vi "鼠标位置.vi"() -> ()   [LabVIEW 2015]
panel:
  out "索引":i32
  out "数组":dbl[][](array[numeric])
  in  "停止":bool
  out "垂直":dbl
  out "水平":dbl
  # "坐标"
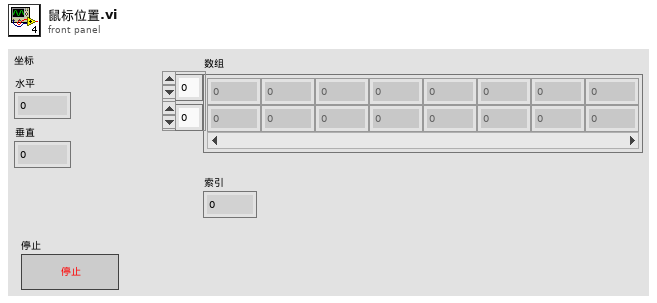
[diagram p1: front panel]
types:
  T1 = typedef "LVPoint32TypeDef.ctl" = cluster{"Horizontal":i32, "Vertical":i32}
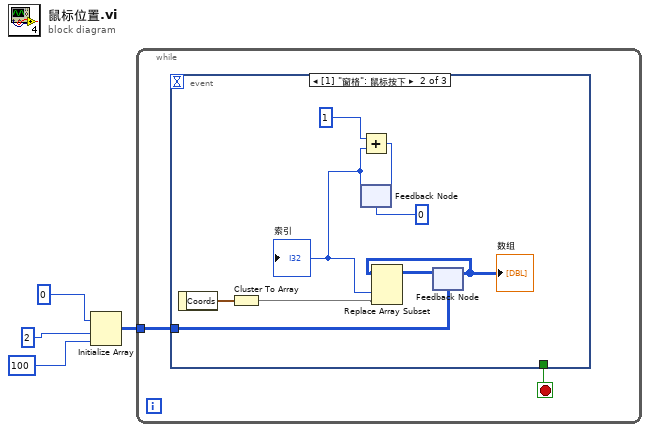
[diagram p0: block diagram]
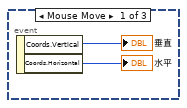
[diagram p2: hidden frame]
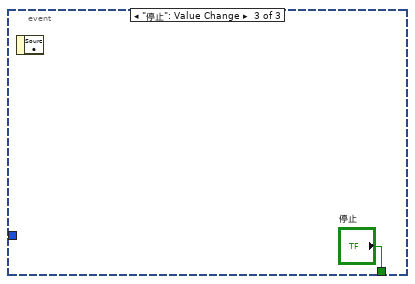
[diagram p3: hidden frame]
diagram:
  n1 = Initialize Array(0, 2, 100) -> (w1:i32[][])
  n2 = while {
    tunnel: w1 -> [w5]
    stop <- w6 stop-if-true
    n3 = event shown="[1] \"窗格\": 鼠标按下" {
      selector: _ -> [_ _ _]
      dyn-events: _ -> [_ _ _]
      timeout: _ -> [_ _ _]
      tunnel: [_ _ "停止"] -> w6
      tunnel: w5 -> [_ w9 _]
      event Mouse Move {
        n4 = event-data() -> ("Coords.Vertical"=→"垂直":i32, "Coords.Horizontal"=→"水平":i32)  [unwired: 1 in]
      }
      event Mouse Down {
        n5 = event-data() -> ("Coords"=w17:T1)  [unwired: 1 in]
        n6 = Cluster To Array(cluster=w17) -> (array=w12:i32[])
        n7 = feedback #1(0) -> (w13:i32)
        "索引" <- w13
        n8 = Add(x=1, y=w13) -> (x+y=w15:i32)
        n9 = feedback-in #1(w15) -> ()
        n10 = feedback #2(w9) -> (w10:i32[][])
        "数组" <- w10
        n11 = Replace Array Subset(array=w10, new element=w12, index (col)=w13) -> (w11:i32[][])  [unwired: 1 in]
        n12 = feedback-in #2(w11) -> ()
      }
      event "停止": Value Change {
        n13 = event-data() -> ()  [unwired: 1 in, 1 out]
      }
    }
  }
